vi "Config Read.vi"(7 "Section":string, 8 "error in (no error)":errorcluster, 10 "Key Names ([]=All Keys)":string[](array[string]), 11 "Path (*.ini) in":path) -> (0 "error out":errorcluster, 1 "Values":string[](array[string]), 2 "Key Names":string[](array[string]), 3 "Path out":path, 4 "Found":bool[](array[boolean]))   [LabVIEW 2022 SP3, in "Core.lvlib"]
uses:
  Core.lvlib
  <vilib>/Utility/config.llb/Read Key (String).vi
  <vilib>/Utility/config.llb/NI_LVConfig.lvlib
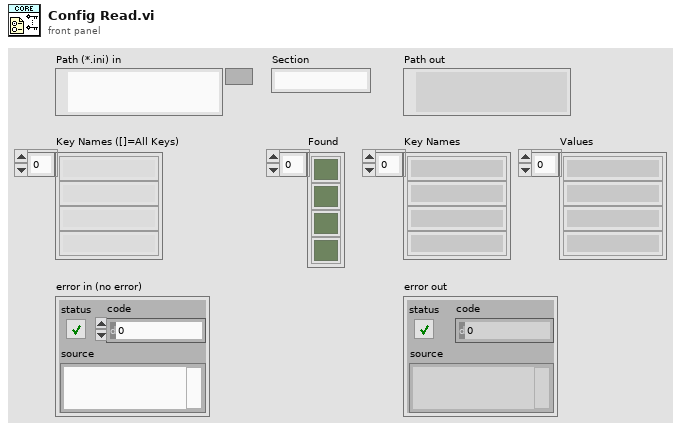
[diagram p1: front panel]
types:
  T1 = typedef "NI_LVConfig.lvlib/Config Data RefNum.ctl" = refnum<k1>
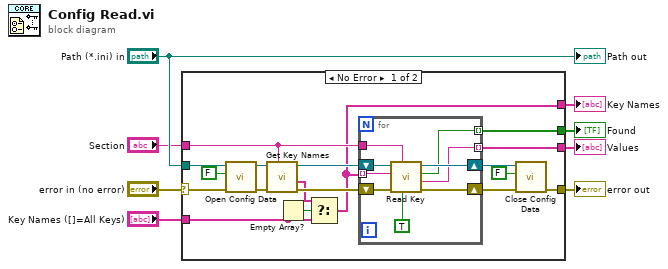
[diagram p0: block diagram]
diagram:
  n1 = case shown="No Error" "error in (no error)" {
    selector: "error in (no error)" -> [w16 w36]
    tunnel: "Path (*.ini) in" -> [w18 _]
    tunnel: "Section" -> [w17 _]
    tunnel: [w15 w36] -> w5
    tunnel: [w14 _] -> w4
    tunnel: [w13 _] -> w3
    tunnel: "Key Names ([]=All Keys)" -> [w11 _]
    tunnel: [w9 _] -> w1
    frame No Error {
      n2 = call <vilib>:"Open Config Data.vi"("error in (no error)"=w16, "create file if necessary (T)"=FALSE, "configuration file path"=w18) -> ("error out"=w26:errorcluster, "refnum"=w25:T1)  [unwired: 6 in, 1 out]
      n3 = call <vilib>:"Get Key Names.vi"("section"=w17, "error in (no error)"=w26, "refnum"=w25) -> ("error out"=w24:errorcluster, "key names"=w10:string[], "refnum out"=w23:T1)  [unwired: 5 in, 1 out]
      n4 = Empty Array?(array=w11) -> (empty?=w12:bool)
      n5 = Select(t=w10, s=w12, f=w11) -> (s? t:f=w9:string[])
      n6 = for {
        shift-right: [w32] -> w21
        shift-left: w24 -> [w35]
        shift-right: [w33] -> w22
        shift-left: w23 -> [w34]
        tunnel: w9 -> [w30] mode=indexing
        tunnel: w17 -> [w29]
        tunnel: [w28] -> w14 mode=indexing
        tunnel: [w27] -> w13 mode=indexing
        n7 = call-poly <vilib>:"Read Key.vi"("read raw string? (F)"=TRUE, "section"=w29, "error in (no error)"=w35, "key"=w30, "refnum"=w34) -> ("error out"=w32:errorcluster, "value"=w28:string, "found?"=w27:bool, "refnum out"=w33:T1)  [unwired: 3 in]
      }
      n8 = call <vilib>:"Close Config Data.vi"("error in (no error)"=w21, "write file if changed (T)"=FALSE, "refnum"=w22) -> ("error out"=w15:errorcluster)  [unwired: 7 in, 1 out]
    }
    frame Error {
    }
  }
  "error out" <- w5
  "Key Names" <- w1
  "Values" <- w4
  "Found" <- w3
  "Path out" <- "Path (*.ini) in"
